vi "_PassAllowedMessage - MsgList.vi"(5 "Allowed Message":string[](array[string]), 8 "JKISM External Event":string) -> (2 "States":string)   [LabVIEW 2017, in "_csmlite.lvlib"]
uses:
  _csmlite.lvlib
  Communicable State Machine.lvlib
  _Shared/CSM Shared.lvlib
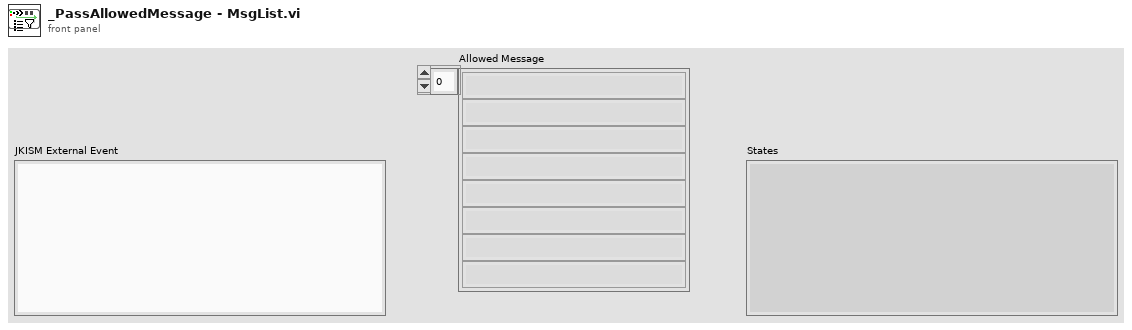
[diagram p1: front panel]
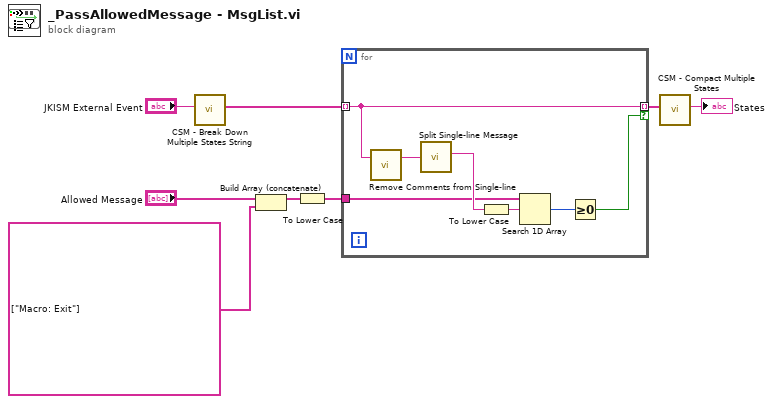
[diagram p0: block diagram]
diagram:
  n1 = call "CSM - Break Down Multiple States String.vi"("States"="JKISM External Event") -> ("Multiple States"=w4:string[])  [unwired: 10 in]
  n2 = Build Array (concatenate)("Allowed Message", string[] ["Macro: Exit"] ("element")) -> (w3:string[])
  n3 = To Lower Case(string=w3) -> (all lower case string=w2:string[])
  n4 = for {
    tunnel: w4 -> [w9] mode=indexing
    tunnel: [w9] -> w6 mode=indexing if=w10
    tunnel: w2 -> [w13]
    n5 = call "Remove Comments from Single-line.vi"("single-line text"=w9) -> ("single-line text without comments"=w15:string)  [unwired: 2 in]
    n6 = call "Split Single-line Message.vi"("single-line text"=w15) -> ("state"=w14:string)  [unwired: 6 in, 3 out]
    n7 = To Lower Case(string=w14) -> (all lower case string=w12:string)
    n8 = Search 1D Array(1D array=w13, element=w12) -> (index of element=w11:i32)  [unwired: 1 in]
    n9 = Greater Or Equal To 0?(x=w11) -> (x >= 0?=w10:bool)
  }
  n10 = call "CSM - Compact Multiple States.vi"("Multiple States"=w6) -> ("States"=→"States":string)  [unwired: 9 in]
